vi "example_read_device_info.vi"() -> ()   [LabVIEW 2012]
doc: "EXAMPLE: Get Device Information\n\nThis example VI retrieves both Device ID and Product ID of the device at the given index. If only one device is connected, that device's index is '0'.\n\nProduced By:\n\nChristopher Lemieux\nKod Integrations, LLC\n4835 Marianne Drive\nMount Airy, MD 21771\nhttp://www.kodintegrations.com\nemail: clemieux@kodintegrations.com\nphone: (240) 687-1288"
uses:
  main_functions/commands.ctl
panel:
  in  "device_index (def=0)":i32
  out "Product ID":string
  out "Device ID":string
  out "error out":errorcluster
  in  "error in (no error)":errorcluster
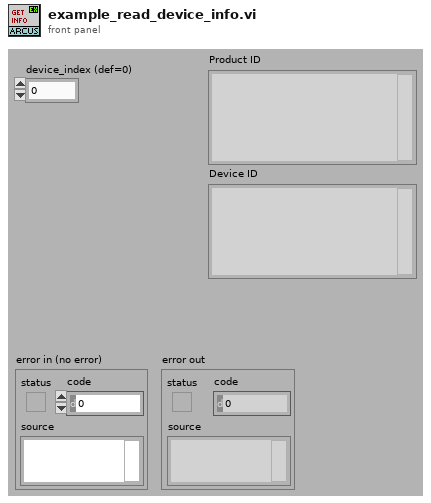
[diagram p1: front panel]
types:
  T1 = typedef "commands.ctl" = enum16{"clearErr", "constJogNeg", "constJogPos", "getAccel", "getActualAmp", "getDeviceId", "getDigInputStatus", "getDigInputsStatus", "getDigOutputStatus", "getDigOutputsStatus", "getFirmwareVer", "getHighSpeed", "getIdleAmp", "getLowSpeed", "getMicroStep", "getMotorStatus", "getMoveMode", "getPolarity", "getPosition", "getProdId", "getPwrStatus", "getRunAmp", "getStatus", "homeNeg", "homePos", "moveToPosition", "powerDown", "powerUp", "setAccel", "setDeviceId", "setDigOutput", "setDigOutputs", "setHighSpeed", "setIdleAmp", "setLowSpeed", "setMoveModeAbs", "setMoveModeIncr", "setPolarity", "setPosition", "setRunAmp", "stopNow", "stopSlow", "storeToMem"}
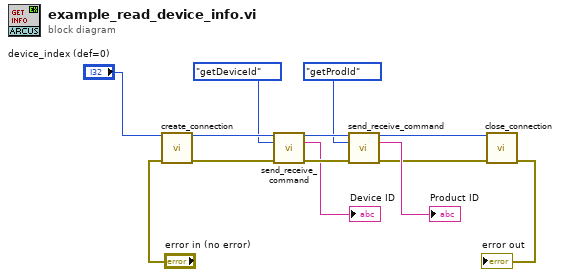
[diagram p0: block diagram]
diagram:
  n1 = call "create_connection.vi"("device_index (def=0)"="device_index (def=0)", "error in (no error)"="error in (no error)") -> ("reference"=w13:i32, "error out"=w11:errorcluster)  [unwired: 12 in]
  n2 = call "send_receive_command.vi"("reference (in)"=w13, "command"=commands."getDeviceId", "error in (no error)"=w11) -> ("reference (dup)"=w10:i32, "read_string"=→"Device ID":string, "error out"=w9:errorcluster)  [unwired: 8 in, 2 out]
  n3 = call "send_receive_command.vi"("reference (in)"=w10, "command"=commands."getProdId", "error in (no error)"=w9) -> ("reference (dup)"=w5:i32, "read_string"=→"Product ID":string, "error out"=w4:errorcluster)  [unwired: 8 in, 2 out]
  n4 = call "close_connection.vi"("reference"=w5, "error in (no error)"=w4) -> ("error out"=→"error out":errorcluster)  [unwired: 13 in]
